vi "Set Register LUT--Accessor.vi"(8 "error in (no error)":errorcluster, 10 "Register LUT":variant, 11 "Watlow F4T in":refnum<class "Watlow F4T.lvclass">) -> (0 "error out":errorcluster, 3 "Watlow F4T out":refnum<class "Watlow F4T.lvclass">)   [LabVIEW 2024, in "Watlow F4T.lvclass"]
uses:
  Watlow F4T.lvclass
  Watlow F4T.lvclass/Watlow F4T.ctl
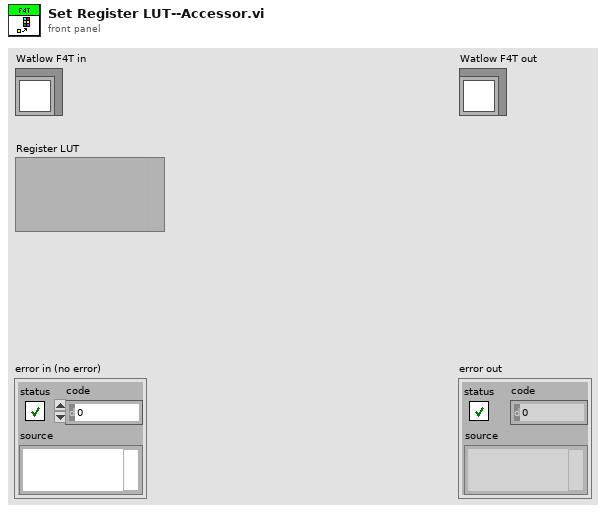
[diagram p1: front panel]
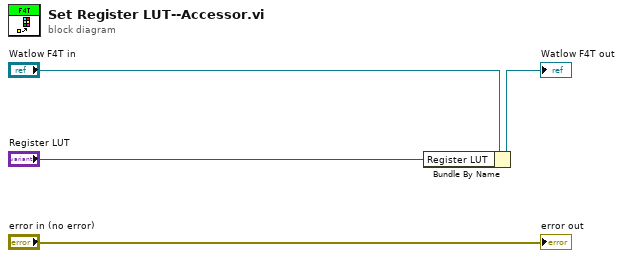
[diagram p0: block diagram]
diagram:
  n1 = Bundle By Name(cluster="Watlow F4T in", "Register LUT"="Register LUT") -> (→"Watlow F4T out":refnum<class "Watlow F4T.lvclass">)
  "error out" <- "error in (no error)"
